vi "Set Camera.vi"(8 "error in (no error)":errorcluster, 10 "Camera":T1, 11 "FormulaG API in":refnum<class "FormulaG API.lvclass">) -> (0 "error out":errorcluster, 3 "FormulaG API out":refnum<class "FormulaG API.lvclass">)   [LabVIEW 2024, in "FormulaG.lvlib" / "FormulaG API.lvclass"]
uses:
  FormulaG API.lvclass
  FormulaG-Common/Camera.ctl
  Command.ctl
  FormulaG API.lvclass/FormulaG API.ctl
  <vilib>/IlluminatedG/IG GodotServer/GodotLV/GodotServer/GodotServer.lvclass
  FormulaG-Common/FormulaG-Common.lvlib
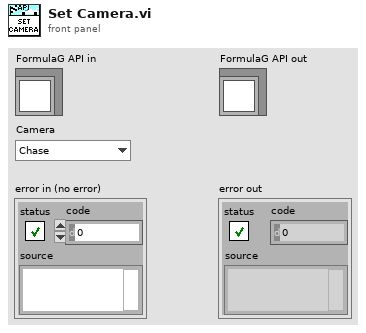
[diagram p1: front panel]
types:
  T1 = typedef "FormulaG-Common.lvlib/Camera.ctl" = enum16{"Chase", "Overhead"}
  T2 = enum16{"big-endian, network order", "native, host order", "little-endian"}
  T3 = typedef "FormulaG.lvlib/FormulaG API.lvclass/Command.ctl" = enum8{"None", "Reset Car", "Request State", "Control Car", "Request Info", "Set Options", "Set Camera", "Set Pause", "Request Time"}
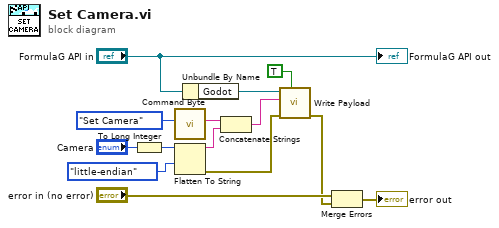
[diagram p0: block diagram]
diagram:
  n1 = To Long Integer(number="Camera") -> (32bit integer=w7:i32)
  n2 = call "Command Byte.vi"("Command"=Command."Set Camera") -> ("Command Byte"=w11:string)  [unwired: 10 in]
  n3 = Flatten To String(anything=w7, byte order (0:big-endian, network order)=T2."little-endian") -> (data string=w5:string, error out=w4:errorcluster)  [unwired: 2 in, 1 out]
  n4 = Unbundle By Name("FormulaG API in") -> ("Godot"=w10:refnum<class "GodotServer.lvclass">)
  n5 = Concatenate Strings(w11, w5) -> (w9:string)
  n6 = call <vilib>:"Write Payload.vi"("Binary (F = Text)"=TRUE, "error in (no error)"=w4, "Payload"=w9, "GodotServer in"=w10) -> ("error out"=w2:errorcluster)  [unwired: 6 in, 1 out]
  n7 = Merge Errors("error in (no error)", w2) -> (→"error out":errorcluster)
  "FormulaG API out" <- "FormulaG API in"
